vi "Mult Enable queue.vi"(8 "error in":errorcluster, 10 "Command":T1[](array[typedef]), 11 "queue in":refnum<queue>) -> (0 "error out":errorcluster, 3 "queue out":refnum<queue>)   [LabVIEW 2017]
uses:
  controls/QI_6251ai.ctl
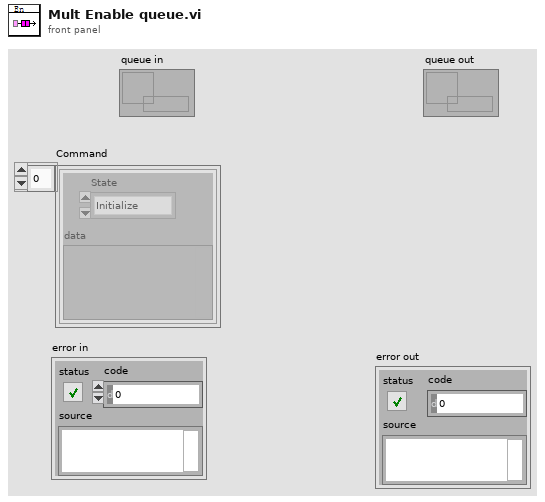
[diagram p1: front panel]
types:
  T1 = typedef "QI_6251ai.ctl" = cluster{"State":enum16{"Initialize", "Mode chang", "Start acquire", "Read data", "Stop acquire"}, "data":variant}
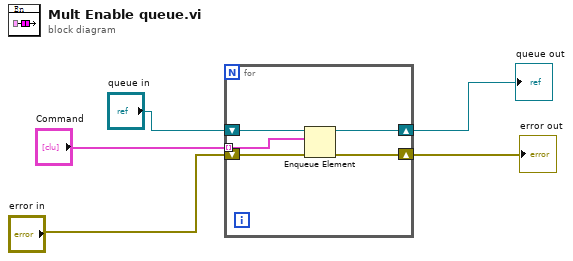
[diagram p0: block diagram]
diagram:
  n1 = for {
    shift-right: [w10] -> w5
    shift-left: "error in" -> [w9]
    shift-right: [w8] -> w1
    shift-left: "queue in" -> [w7]
    tunnel: "Command" -> [w6] mode=indexing
    n2 = Enqueue Element(queue=w7, element=w6, error in (no error)=w9) -> (queue out=w8:refnum<queue>, error out=w10:errorcluster)  [unwired: 1 in, 1 out]
  }
  "error out" <- w5
  "queue out" <- w1
